vi "Login-Window.vi"(8 "Error in":errorcluster caption="Error in (no error)", 11 "Options":cluster{"HideMain(T)":bool}={"HideMain(T)"=TRUE}) -> (0 "Error out":errorcluster={"status"=TRUE, "code"=43, "source"="Operation cancelled by user."}, 1 "Valid User":bool, 3 "User Info":T1)   [LabVIEW 2020]
uses:
  Typedef/User-Info.ctl
  Typedef/User-Role.ctl
  _support/_password_db_oper.ctl
  82dbac5f-f66d-497b-81a9-0f95a8baf484.vi
panel:
  in  "UserManage":bool
  in  "Login":bool
  in  "Password":string="admin" caption="密  码"
  in  "UserName":string="admin" caption="用户名"
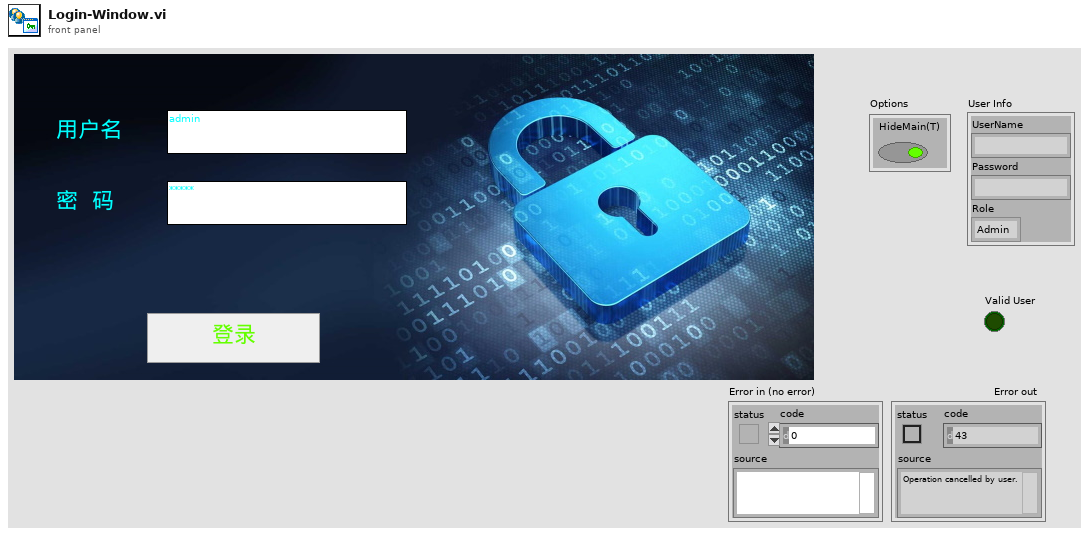
[diagram p1: front panel]
types:
  T1 = typedef "User-Info.ctl" = cluster{"UserName":string, "Password":string, "Role":T2}
  T2 = typedef "User-Role.ctl" = enum16{"Admin", "Engineer", "Operator"}
  T3 = enum32{"Invalid", "Standard", "Closed", "Hidden", "Minimized", "Maximized"}
  T4 = typedef "_password_db_oper.ctl" = enum16{"Validate", "Register", "Unregister", "View"}
  T5 = typedef "eventvkey.ctl" = enum16{"ASCII", "Enter", "Return", "Shift", "Ctrl", "Alt", "Cmd", "Opt", "Caps", "NumLock", "Clear", "Break", "Up", "Down", "Left", "Right", "Insert", "Delete", "Home", "End", "PageUp", "PageDown", "Escape", "Help", "Pause", "ScrollLock", "F1", "F2", "F3", "F4", "F5", "F6", "F7", "F8", "F9", "F10", "F11", "F12", "F13", "F14", "F15", "F16", "F17", "F18", "F19", "F20", "F21", "F22", "F23", "F24", "Play", "VolumeUp", "VolumeDown", "Mute", "Two Byte Char"}
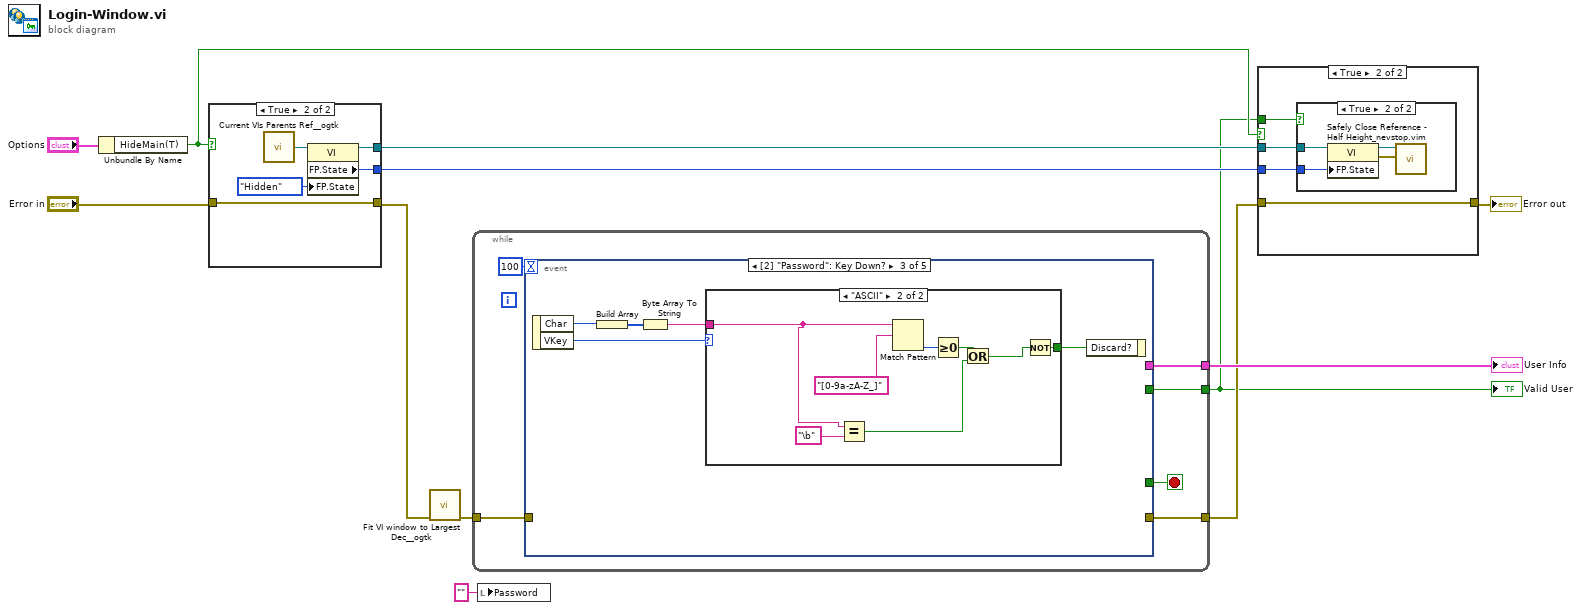
[diagram p0: block diagram]
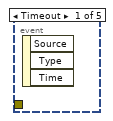
[diagram p5: hidden frame]
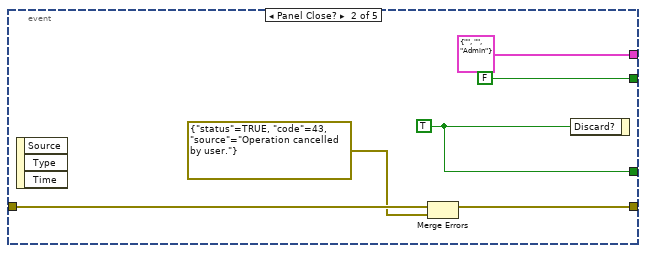
[diagram p6: hidden frame]
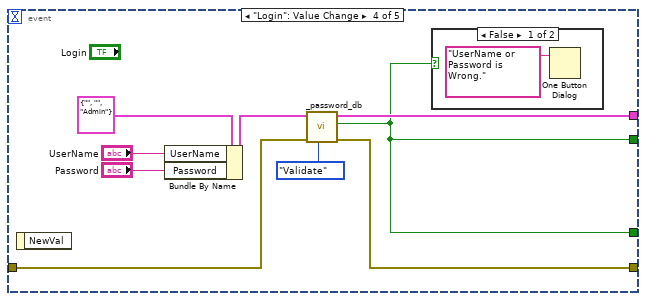
[diagram p8: hidden frame]
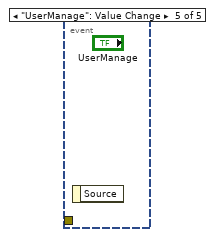
[diagram p10: hidden frame]
diagram:
  n1 = Unbundle By Name("Options") -> ("HideMain(T)"=w5:bool)
  n2 = case shown="True" w5 {
    tunnel: [_ w16] -> w11
    tunnel: [_ w15] -> w10
    tunnel: [w13 w14] -> w7
    tunnel: "Error in" -> [w13 w14]
    frame False {
    }
    frame True {
      n3 = call <userlib>:"Current VIs Parents Ref__ogtk.vi"() -> ("Calling VI's Reference"=w18:refnum<vi>)  [unwired: 2 in]
      n4 = property class="VI"(reference=w18, "FP.State"=T3."Hidden" ("Front Panel Window:State")) -> (reference out=w15:refnum<vi>, "FP.State"=w16:T3)  [unwired: 1 in, 1 out]
    }
  }
  n5 = call <userlib>:"Fit VI window to Largest Dec__ogtk.vi"("error in (no error)"=w7) -> ("error out"=w12:errorcluster)  [unwired: 5 in, 1 out]
  n6 = while {
    tunnel: w12 -> [w20]
    tunnel: [w22] -> w4
    tunnel: [w21] -> w3
    tunnel: [w19] -> w2
    stop <- w24 stop-if-true
    n7 = event shown="[2] \"Password\": Key Down?" {
      selector: _ -> [_ _ _ _ _]
      dyn-events: _ -> [_ _ _ _ _]
      timeout: 100 -> [_ _ _ _ _]
      tunnel: [_ w30 _ w44 _] -> w24
      tunnel: [_ T1 {"UserName"="", "Password"="", "Role"=enum."Admin"} ("User Info") _ w51 _] -> w22
      tunnel: [_ w26 _ w49 _] -> w21
      tunnel: w20 -> [_ w28 _ w50 _]
      tunnel: [_ FALSE ("Discard?") _ w44 _] -> w19
      event Timeout {
        n8 = event-data() -> ()  [unwired: 1 in, 3 out]
      }
      event Panel Close? {
        w30 = TRUE ("Discard?")
        n9 = event-data() -> ()  [unwired: 1 in, 3 out]
        n10 = Merge Errors(w28, errorcluster {"status"=TRUE, "code"=43, "source"="Operation cancelled by user."} ("error in")) -> (w26:errorcluster)
        n11 = event-data("Discard?"=w30) -> ()  [unwired: 1 in, 1 out]
      }
      event "Password": Key Down? {
        n12 = event-data() -> ("Char"=w32:i16, "VKey"=w34:T5)  [unwired: 1 in]
        n13 = Build Array(w32) -> (w33:i16[])
        n14 = Byte Array To String(unsigned byte array=w33) -> (string=w31:string)
        n15 = case shown="\"ASCII\"" w34 {
          tunnel: [_ w36] -> w35
          tunnel: w31 -> [_ w39]
          frame Default {
          }
          frame "ASCII" {
            n16 = Equal?(x=w39, y="\b" ("regular expression")) -> (x = y?=w37:bool)
            n17 = Match Pattern(string=w39, regular expression="[0-9a-zA-Z_]") -> (offset past match=w42:i32)  [unwired: 1 in, 3 out]
            n18 = Greater Or Equal To 0?(x=w42) -> (x >= 0?=w41:bool)
            n19 = Or(x=w41, y=w37) -> (x .or. y?=w38:bool)
            n20 = Not(x=w38) -> (.not. x?=w36:bool)
          }
        }
        n21 = event-data("Discard?"=w35) -> ()  [unwired: 1 in, 1 out]
      }
      event "Login": Value Change {
        n22 = event-data() -> ()  [unwired: 1 in, 1 out]
        n23 = Bundle By Name(cluster=T1 {"UserName"="", "Password"="", "Role"=enum."Admin"} ("Userinfo"), "UserName"="UserName", "Password"="Password") -> (w47:T1)
        n24 = call "_password_db.vi"("Enum"=_password_db_oper."Validate", "Error in"=w50, "Userinfo"=w47) -> ("Error out"=w49:errorcluster, "Boolean"=w44:bool, "Userinfo (dup)"=w51:T1)  [unwired: 6 in]
        n25 = case shown="False" w44 {
          frame False {
            n26 = One Button Dialog(message="UserName or Password is Wrong.") -> ()  [unwired: 1 in, 1 out]
          }
          frame True {
          }
        }
      }
      event "UserManage": Value Change {
        n27 = event-data() -> ()  [unwired: 1 in, 1 out]
      }
    }
  }
  "User Info" <- w4
  "Valid User" <- w2
  n28 = local write "Password"("" ("Password")) -> ()
  n29 = case shown="True" w5 {
    tunnel: w11 -> [_ w58]
    tunnel: w10 -> [_ w57]
    tunnel: [w54 w56] -> w8
    tunnel: w3 -> [w54 w56]
    tunnel: w2 -> [_ w55]
    frame False {
    }
    frame True {
      n30 = case shown="True" w55 {
        tunnel: w58 -> [_ w62]
        tunnel: w57 -> [_ w61]
        frame False {
        }
        frame True {
          n31 = property class="VI"(reference=w61, "FP.State"=w62) -> (reference out=w59:refnum<vi>, error out=w60:errorcluster)  [unwired: 1 in]
          n32 = call "Safely Close Reference - Half Height_nevstop.vim"("error in (no error)"=w60, "Reference"=w59) -> ()  [unwired: 9 in, 1 out]
        }
      }
    }
  }
  "Error out" <- w8
